vi "test_maj_ASIC.vi"() -> ()   [LabVIEW 2009]
uses:
  <vilib>/Utility/NIReport.llb/NI_report.lvclass
  <vilib>/Utility/NIReport.llb/HTML/NI_HTML.lvclass
panel:
  in  "threshold":i32[][](array[numeric])
  in  "Sums":bool=TRUE
  in  "Full test":bool=TRUE
  out "error out":errorcluster
  out "Instrument VISA out":T1={"AWG VISA"="generadorpulsos", "Oscilloscope  VISA "="Oscilloscope", "Integration Board IP"="172.16.7.43", "connection ID"=refnum, "report out"=refnum, "report file path"=path "D:/CTA/Data_test/ASIC/test3a"}
  in  "Save NOW!":bool
  in  "Instrument VISA in":T1={"AWG VISA"="generadorpulsos", "Oscilloscope  VISA "="Oscilloscope", "Integration Board IP"="172.16.7.43", "connection ID"=refnum, "report out"=refnum, "report file path"=path "D:/CTA/Data_test/ASIC/chip_test"}
  in  "error in":errorcluster
  in  "Channels":i32[](array[numeric])=[0, 1, 2, 3, 4, 5, 6]
  in  "Voltages comprobation":dbl[](array[numeric])=[0.05, 0.1, 0.2, 0.3, 0.4, 0.5, 0.6, 0.7, 0.8, 1.0]
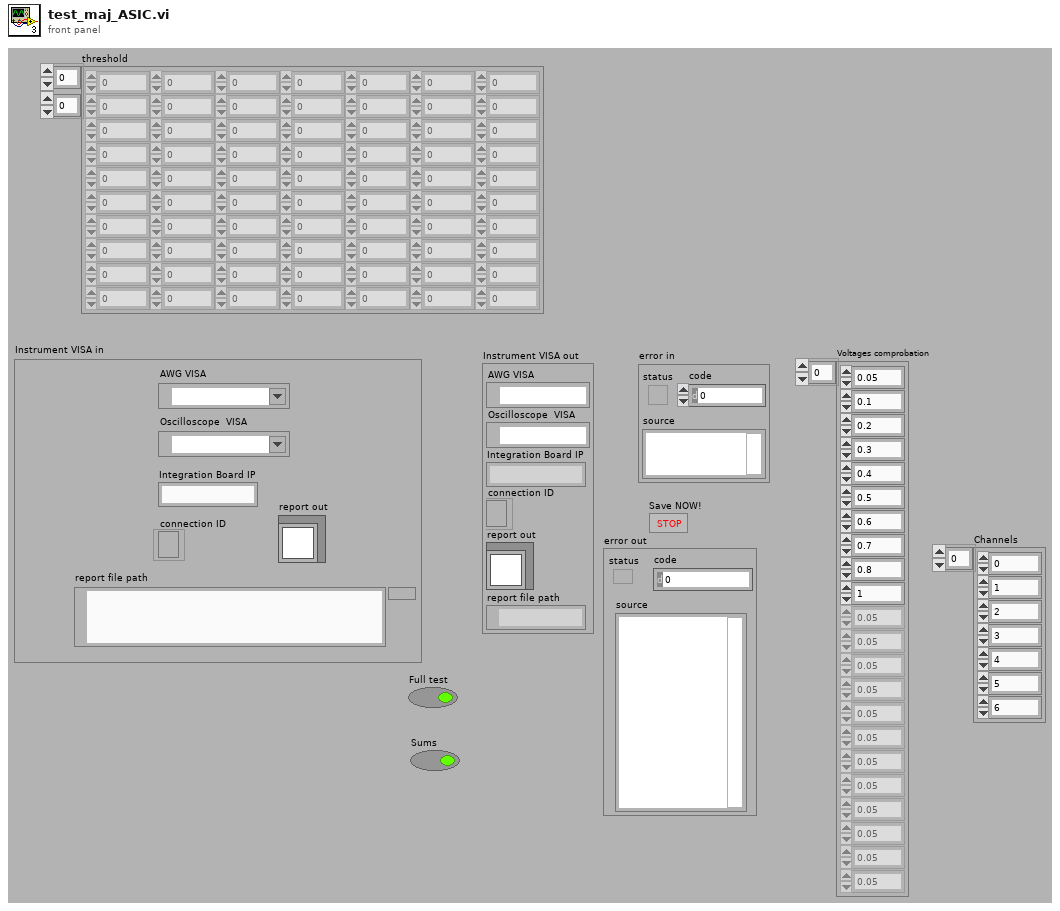
[diagram p1: front panel]
types:
  T1 = cluster{"AWG VISA":refnum<visa-resource-name>, "Oscilloscope  VISA ":refnum<visa-resource-name>, "Integration Board IP":string, "connection ID":refnum<k5>, "report out":refnum<class "NI_report.lvclass">, "report file path":path}
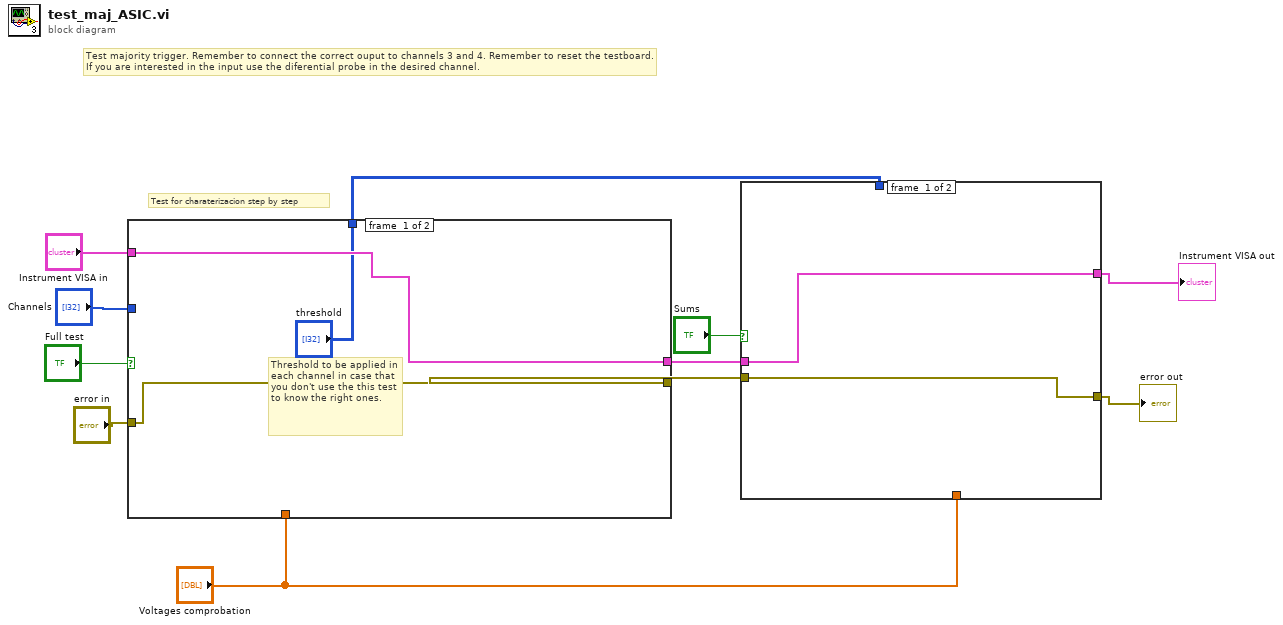
[diagram p0: block diagram]
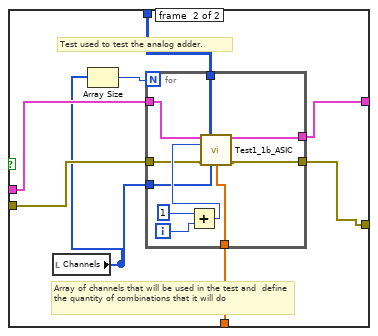
[diagram p2: hidden frame]
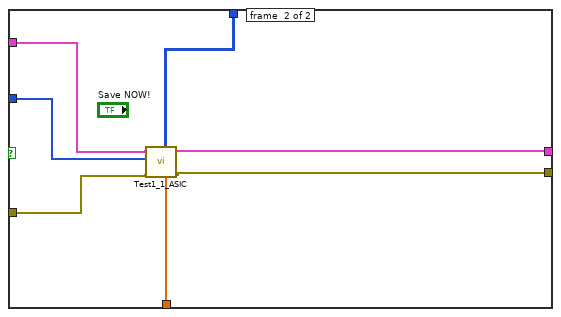
[diagram p3: hidden frame]
diagram:
  # "Test for charaterizacion step by step"
  # "Test majority trigger. Remember to connect the correct ouput to channels 3 and 4. Remember to reset the testboard. \nIf you are interested in the input use the diferential probe in the desired channel."
  n1 = case shown="True" "Full test" {
    tunnel: "Voltages comprobation" -> [_ w17]
    tunnel: "error in" -> [w14 w19]
    tunnel: "Channels" -> [_ w16]
    tunnel: "Instrument VISA in" -> [w13 w18]
    tunnel: [w14 w20] -> w2
    tunnel: [w13 w21] -> w1
    tunnel: ["threshold" w15] -> w4
    frame #0 {
      # "Threshold to be applied in each channel in case that you don't use the this test to know the right ones."
    }
    frame #1 {
      n2 = call "Test1_1_ASIC.vi"("Voltages comprobation"=w17, "error in"=w19, "Channels"=w16, "Instrument VISA in"=w18) -> ("error out"=w20:errorcluster, "Instrument VISA out"=w21:T1, "Array"=w15:i32[][])  [unwired: 5 in]
    }
  }
  n3 = case shown="True" "Sums" {
    tunnel: [w22 w31] -> w8
    tunnel: [w23 w29] -> w9
    tunnel: w2 -> [w23 w30]
    tunnel: w1 -> [w22 w28]
    tunnel: w4 -> [_ w25]
    tunnel: "Voltages comprobation" -> [_ w24]
    frame #0 {
    }
    frame #1 {
      # "Test used to test the analog adder."
      # "Array of channels that will be used in the test and  define the quantity of combinations that it will do"
      n4 = local read "Channels"() -> (w27:i32[])
      n5 = Array Size(array=w27) -> (size(s)=w26:i32)
      n6 = for {
        N: w26 -> [_]
        tunnel: [w40] -> w31
        tunnel: w28 -> [w39]
        tunnel: w30 -> [w37]
        tunnel: [w36] -> w29
        tunnel: w27 -> [w35]
        tunnel: w25 -> [w33]
        tunnel: w24 -> [w32]
        i -> [w41]
        n7 = Add(x=1 ("y"), y=w41) -> (x+y=w38:i32)
        n8 = call "Test1_1b_ASIC.vi"("Instrument VISA in"=w39, "threshold"=w33, "quantity"=w38, "error in"=w37, "channel array"=w35, "Voltages comprobation"=w32) -> ("Instrument VISA out"=w40:T1, "error out"=w36:errorcluster)  [unwired: 8 in]
      }
    }
  }
  "Instrument VISA out" <- w8
  "error out" <- w9
